vi "Create_Raw_data_folder.vi"(1 "Folder Name":string="Paul:DispC", 3 "Data Type":string="Colour Calib") -> (0 "Raw Data Folder":path)   [LabVIEW 2011]
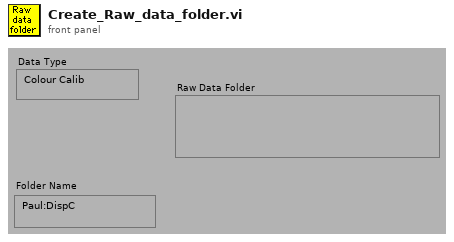
[diagram p1: front panel]
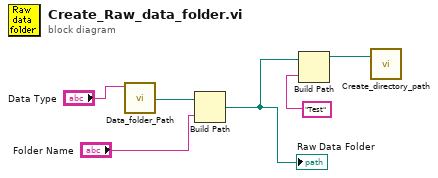
[diagram p0: block diagram]
diagram:
  n1 = call "Data_folder_Path.vi"("Data Type"="Data Type") -> ("Data Folder"=w3:path)  [unwired: 4 in]
  n2 = Build Path(base path=w3, name or relative path="Folder Name") -> (appended path=w1:path)
  "Raw Data Folder" <- w1
  n3 = Build Path(base path=w1, name or relative path="Test" ("Substring")) -> (appended path=w5:path)
  n4 = call "Create_directory_path.vi"("Path name"=w5) -> ()  [unwired: 1 in, 2 out]
